vi "aggregate data.vi"() -> ()   [LabVIEW 2020]
panel:
  out "dG/dt/G vs temp hrs":cluster{"Data":dbl[], "Data":dbl[]}[](graph)
  out "dG/dt/G vs temp":cluster{"Data":dbl[], "Data":dbl[]}[](graph)
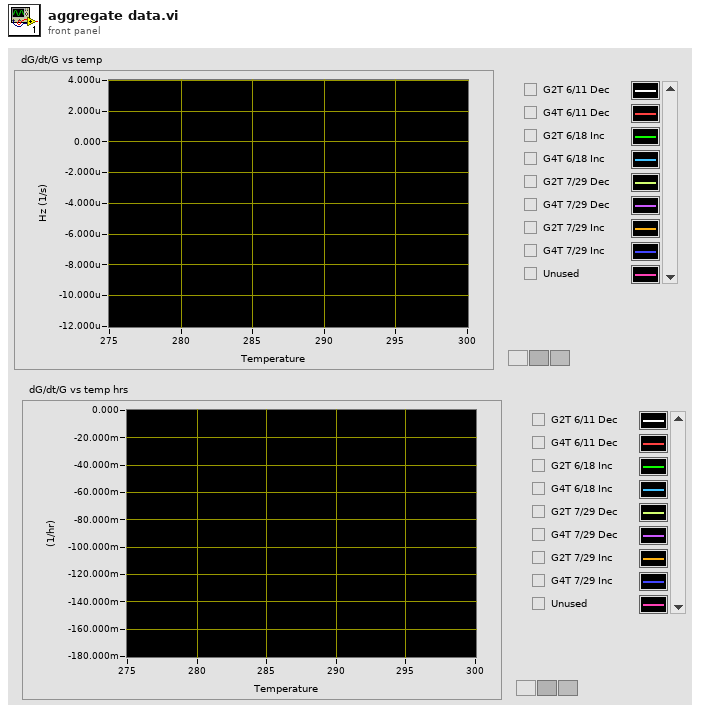
[diagram p1: front panel]
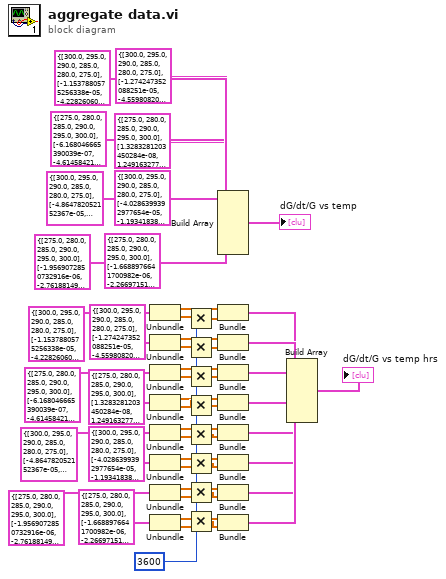
[diagram p0: block diagram]
diagram:
  w34 = 3600
  n1 = Unbundle(cluster{dbl[], dbl[]} {[300.0, 295.0, 290.0, 285.0, 280.0, 275.0], [-1.1537880575256338e-05, -4.22826060820674e-06, -2.3653742417541264e-06, -1.3028566769234502e-06, -7.890287594859811e-07, -4.7153090154693677e-07]}) -> (w10:dbl[], w19:dbl[])
  n2 = Unbundle(cluster{dbl[], dbl[]} {[300.0, 295.0, 290.0, 285.0, 280.0, 275.0], [-1.274247352088251e-05, -4.55980820011919e-06, -2.5020592499196788e-06, -1.3489355716779094e-06, -7.925451445036797e-07, -4.908004729274311e-07]}) -> (w11:dbl[], w21:dbl[])
  n3 = Unbundle(cluster{dbl[], dbl[]} {[275.0, 280.0, 285.0, 290.0, 295.0, 300.0], [-6.168046665390039e-07, -4.614584211590721e-07, -9.919628619405374e-07, -1.1729746337105461e-06, -1.4549767203751042e-06, -1.4669053747807315e-06]}) -> (w12:dbl[], w23:dbl[])
  n4 = Unbundle(cluster{dbl[], dbl[]} {[275.0, 280.0, 285.0, 290.0, 295.0, 300.0], [1.3283281203450284e-08, 1.2491632770265845e-06, 2.377655533158304e-06, 3.240051016739081e-06, 2.3491507311046513e-06, -3.288238336519177e-07]}) -> (w13:dbl[], w25:dbl[])
  n5 = Unbundle(cluster{dbl[], dbl[]} {[300.0, 295.0, 290.0, 285.0, 280.0, 275.0], [-4.864782052152367e-05, -1.4394380255731984e-05, -7.063298030319999e-06, -4.797818894900328e-06, -3.0858711624502367e-06, -2.185253068975472e-06]}) -> (w14:dbl[], w27:dbl[])
  n6 = Unbundle(cluster{dbl[], dbl[]} {[300.0, 295.0, 290.0, 285.0, 280.0, 275.0], [-4.0286399392977654e-05, -1.1934183863055551e-05, -5.895450541703924e-06, -3.85186272225402e-06, -2.6126636167088024e-06, -1.8906421875696023e-06]}) -> (w15:dbl[], w29:dbl[])
  n7 = Unbundle(cluster{dbl[], dbl[]} {[275.0, 280.0, 285.0, 290.0, 295.0, 300.0], [-1.9569072850732916e-06, -2.761881494172482e-06, -4.449507739391446e-06, -6.177357233872075e-06, -8.712607839906274e-06, -1.0760041167626922e-05]}) -> (w16:dbl[], w31:dbl[])
  n8 = Unbundle(cluster{dbl[], dbl[]} {[275.0, 280.0, 285.0, 290.0, 295.0, 300.0], [-1.6688976641700982e-06, -2.266971514382747e-06, -3.50807439271461e-06, -4.982535821006548e-06, -6.8843627012033555e-06, -8.4429552355069e-06]}) -> (w17:dbl[], w33:dbl[])
  n9 = Multiply(x=w19, y=w34) -> (x*y=w18:dbl[])
  n10 = Multiply(x=w21, y=w34) -> (x*y=w20:dbl[])
  n11 = Multiply(x=w23, y=w34) -> (x*y=w22:dbl[])
  n12 = Multiply(x=w25, y=w34) -> (x*y=w24:dbl[])
  n13 = Multiply(x=w27, y=w34) -> (x*y=w26:dbl[])
  n14 = Multiply(x=w29, y=w34) -> (x*y=w28:dbl[])
  n15 = Multiply(x=w31, y=w34) -> (x*y=w30:dbl[])
  n16 = Multiply(x=w33, y=w34) -> (x*y=w32:dbl[])
  n17 = Build Array(cluster{dbl[], dbl[]} {[300.0, 295.0, 290.0, 285.0, 280.0, 275.0], [-1.1537880575256338e-05, -4.22826060820674e-06, -2.3653742417541264e-06, -1.3028566769234502e-06, -7.890287594859811e-07, -4.7153090154693677e-07]}, cluster{dbl[], dbl[]} {[300.0, 295.0, 290.0, 285.0, 280.0, 275.0], [-1.274247352088251e-05, -4.55980820011919e-06, -2.5020592499196788e-06, -1.3489355716779094e-06, -7.925451445036797e-07, -4.908004729274311e-07]}, cluster{dbl[], dbl[]} {[275.0, 280.0, 285.0, 290.0, 295.0, 300.0], [-6.168046665390039e-07, -4.614584211590721e-07, -9.919628619405374e-07, -1.1729746337105461e-06, -1.4549767203751042e-06, -1.4669053747807315e-06]}, cluster{dbl[], dbl[]} {[275.0, 280.0, 285.0, 290.0, 295.0, 300.0], [1.3283281203450284e-08, 1.2491632770265845e-06, 2.377655533158304e-06, 3.240051016739081e-06, 2.3491507311046513e-06, -3.288238336519177e-07]}, cluster{dbl[], dbl[]} {[300.0, 295.0, 290.0, 285.0, 280.0, 275.0], [-4.864782052152367e-05, -1.4394380255731984e-05, -7.063298030319999e-06, -4.797818894900328e-06, -3.0858711624502367e-06, -2.185253068975472e-06]}, cluster{dbl[], dbl[]} {[300.0, 295.0, 290.0, 285.0, 280.0, 275.0], [-4.0286399392977654e-05, -1.1934183863055551e-05, -5.895450541703924e-06, -3.85186272225402e-06, -2.6126636167088024e-06, -1.8906421875696023e-06]}, cluster{dbl[], dbl[]} {[275.0, 280.0, 285.0, 290.0, 295.0, 300.0], [-1.9569072850732916e-06, -2.761881494172482e-06, -4.449507739391446e-06, -6.177357233872075e-06, -8.712607839906274e-06, -1.0760041167626922e-05]}, cluster{dbl[], dbl[]} {[275.0, 280.0, 285.0, 290.0, 295.0, 300.0], [-1.6688976641700982e-06, -2.266971514382747e-06, -3.50807439271461e-06, -4.982535821006548e-06, -6.8843627012033555e-06, -8.4429552355069e-06]}) -> (→"dG/dt/G vs temp":cluster{dbl[], dbl[]}[])
  n18 = Bundle(w10, w18) -> (w2:cluster{dbl[], dbl[]})  [unwired: 1 in]
  n19 = Bundle(w11, w20) -> (w3:cluster{dbl[], dbl[]})  [unwired: 1 in]
  n20 = Bundle(w12, w22) -> (w4:cluster{dbl[], dbl[]})  [unwired: 1 in]
  n21 = Bundle(w13, w24) -> (w5:cluster{dbl[], dbl[]})  [unwired: 1 in]
  n22 = Bundle(w14, w26) -> (w6:cluster{dbl[], dbl[]})  [unwired: 1 in]
  n23 = Bundle(w15, w28) -> (w7:cluster{dbl[], dbl[]})  [unwired: 1 in]
  n24 = Bundle(w16, w30) -> (w8:cluster{dbl[], dbl[]})  [unwired: 1 in]
  n25 = Bundle(w17, w32) -> (w9:cluster{dbl[], dbl[]})  [unwired: 1 in]
  n26 = Build Array(w2, w3, w4, w5, w6, w7, w8, w9) -> (→"dG/dt/G vs temp hrs":cluster{dbl[], dbl[]}[])
